vi "PathDialog.vi"() -> (3 "Cancelled?":bool)   [LabVIEW 2020]
doc: "Use this template to create a dialog box with event handling."
uses:
  global/SettingVariable.vi
  <vilib>/Utility/config.llb/Write Key (Path).vi
  <vilib>/Utility/config.llb/NI_LVConfig.lvlib
panel:
  in  "DRWM path 2":path caption="DRWM下段修正因子："
  in  "DRWM path 1":path caption="DRWM上段修正因子："
  in  "data path":path caption="数据文件保存路径："
  in  "Cancel":bool
  in  "OK":bool
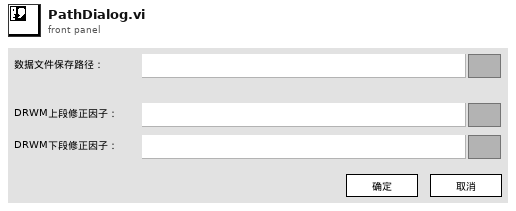
[diagram p1: front panel]
types:
  T1 = typedef "NI_LVConfig.lvlib/Config Data RefNum.ctl" = refnum<k1>
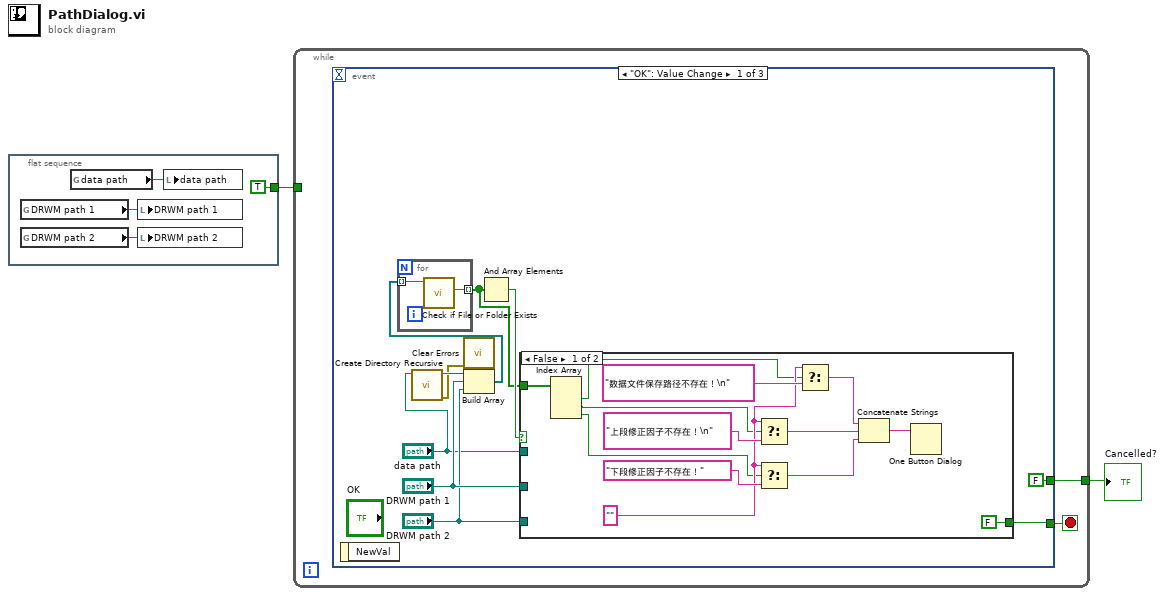
[diagram p0: block diagram]
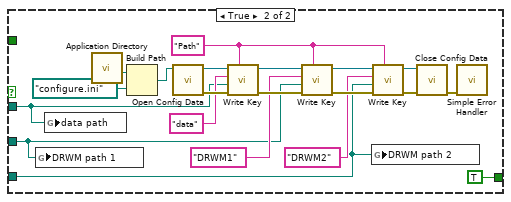
[diagram p2: hidden frame]
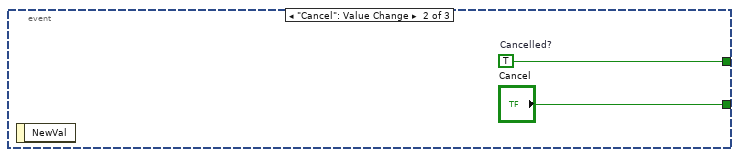
[diagram p3: hidden frame]
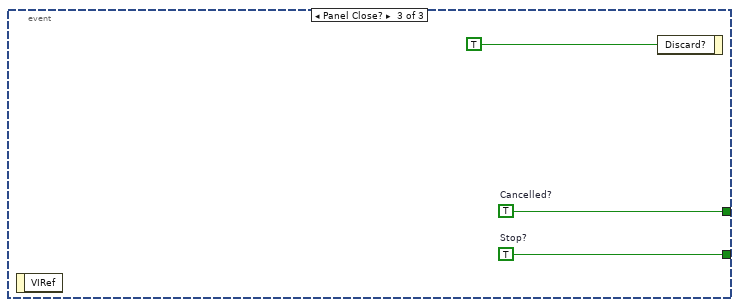
[diagram p4: hidden frame]
diagram:
  n1 = flat-sequence {
    tunnel: [TRUE] -> w1
    frame #0 {
      n2 = global read "SettingVariable.vi" "DRWM path 1"() -> (w5:path)
      n3 = global read "SettingVariable.vi" "DRWM path 2"() -> (w4:path)
      n4 = global read "SettingVariable.vi" "data path"() -> (w6:path)
      n5 = local write "DRWM path 1"(w5) -> ()
      n6 = local write "DRWM path 2"(w4) -> ()
      n7 = local write "data path"(w6) -> ()
    }
  }
  n8 = while {
    tunnel: [w7] -> w2
    tunnel: w1 -> [_]
    stop <- w8 stop-if-true
    n9 = event shown="[0] \"OK\": Value Change" {
      selector: _ -> [_ _ _]
      dyn-events: _ -> [_ _ _]
      timeout: _ -> [_ _ _]
      tunnel: [w17 "Cancel" w57] -> w8
      tunnel: [FALSE ("Cancelled?") w55 w56] -> w7
      event "OK": Value Change {
        n10 = event-data() -> ()  [unwired: 1 in, 1 out]
        n11 = call <vilib>:"Create Directory Recursive.vi"("directory"="data path") -> ("error out"=w9:errorcluster, "directory copy"=w10:path)  [unwired: 4 in, 1 out]
        n12 = call <vilib>:"Clear Errors.vi"("error in (no error)"=w9) -> ()  [unwired: 5 in, 2 out]
        n13 = Build Array(w10, "DRWM path 1", "DRWM path 2") -> (w14:path[])
        n14 = for {
          tunnel: [w20] -> w12 mode=indexing
          tunnel: w14 -> [w19] mode=indexing
          n15 = call <vilib>:"Check if File or Folder Exists.vi"("path"=w19) -> ("file or folder exists?"=w20:bool)  [unwired: 8 in, 2 out]
        }
        n16 = And Array Elements(Boolean array=w12) -> (logical AND=w13:bool)
        n17 = case shown="False" w13 {
          tunnel: [FALSE ("Stop?") TRUE ("Stop?")] -> w17
          tunnel: "data path" -> [_ w36]
          tunnel: "DRWM path 1" -> [_ w35]
          tunnel: "DRWM path 2" -> [_ w34]
          tunnel: w12 -> [w24 _]
          frame False {
            w29 = ""
            n18 = Index Array(array=w24) -> (element #1=w23:bool, element #2=w22:bool, element #3=w21:bool)  [unwired: 3 in]
            n19 = Select(t=w29, s=w22, f="上段修正因子不存在！\n") -> (s? t:f=w27:string)
            n20 = Select(t=w29, s=w21, f="下段修正因子不存在！") -> (s? t:f=w26:string)
            n21 = Select(t=w29, s=w23, f="数据文件保存路径不存在！\n") -> (s? t:f=w28:string)
            n22 = Concatenate Strings(w28, w27, w26) -> (w25:string)
            n23 = One Button Dialog(message=w25) -> ()  [unwired: 1 in, 1 out]
          }
          frame True {
            w43 = "Path" ("section")
            n24 = global write "SettingVariable.vi" "DRWM path 1"(w35) -> ()
            n25 = global write "SettingVariable.vi" "data path"(w36) -> ()
            n26 = call <vilib>:"Application Directory.vi"() -> ("Application Directory"=w52:path)
            n27 = Build Path(base path=w52, name or relative path=path "configure.ini") -> (appended path=w50:path)
            n28 = call <vilib>:"Open Config Data.vi"("configuration file path"=w50) -> ("error out"=w48:errorcluster, "refnum"=w49:T1)  [unwired: 2 in, 7 out]
            n29 = call-poly <vilib>:"Write Key.vi"("section"=w43, "error in (no error)"=w48, "value"=w36, "key"="data" ("section"), "refnum"=w49) -> ("error out"=w46:errorcluster, "refnum out"=w47:T1)  [unwired: 4 in, 1 out]
            n30 = call-poly <vilib>:"Write Key.vi"("section"=w43, "error in (no error)"=w46, "value"=w35, "key"="DRWM1" ("section"), "refnum"=w47) -> ("error out"=w44:errorcluster, "refnum out"=w45:T1)  [unwired: 4 in, 1 out]
            n31 = global write "SettingVariable.vi" "DRWM path 2"(w34) -> ()
            n32 = call-poly <vilib>:"Write Key.vi"("section"=w43, "error in (no error)"=w44, "value"=w34, "key"="DRWM2" ("section"), "refnum"=w45) -> ("error out"=w40:errorcluster, "refnum out"=w41:T1)  [unwired: 4 in, 1 out]
            n33 = call <vilib>:"Close Config Data.vi"("error in (no error)"=w40, "refnum"=w41) -> ("error out"=w42:errorcluster)  [unwired: 1 in, 8 out]
            n34 = call <vilib>:"Simple Error Handler.vi"("error in (no error)"=w42) -> ()  [unwired: 1 in, 8 out]
          }
        }
      }
      event "Cancel": Value Change {
        w55 = TRUE  # Cancelled?
        n35 = event-data() -> ()  [unwired: 1 in, 1 out]
      }
      event Panel Close? {
        w56 = TRUE  # Cancelled?
        w57 = TRUE  # Stop?
        n36 = event-data() -> ()  [unwired: 1 in, 1 out]
        n37 = event-data("Discard?"=TRUE) -> ()  [unwired: 1 in, 1 out]
      }
    }
  }
  "Cancelled?" <- w2
